vi "Trigger Test Harness.vi"() -> ()   [LabVIEW 2014]
panel:
  in  "Boolean":bool
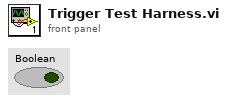
[diagram p1: front panel]
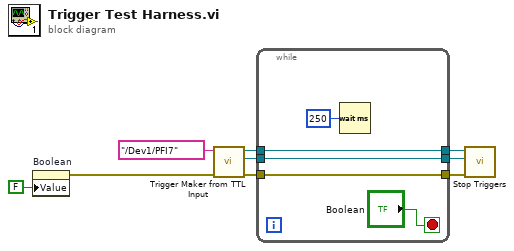
[diagram p0: block diagram]
diagram:
  n1 = property on="Boolean" class="Bool (strict)"("Value"=FALSE ("Boolean")) -> (error out=w1:errorcluster)  [unwired: 2 in, 1 out]
  n2 = call "Trigger Maker from TTL Input.vi"("Error in"=w1, "Master Trigger In from Laser (TTL)"=tag "/Dev1/PFI7") -> ("error out"=w8:errorcluster, "Alazar Task"=w7:refnum<k21>, "AFG11000 Task"=w9:refnum<k21>)  [unwired: 7 in]
  n3 = while {
    tunnel: w9 -> [w13]
    tunnel: w8 -> [w12]
    tunnel: w7 -> [w11]
    tunnel: [w13] -> w5
    tunnel: [w12] -> w4
    tunnel: [w11] -> w3
    stop <- "Boolean" stop-if-true
    n4 = Wait (ms)(milliseconds to wait=u32 250) -> ()  [unwired: 1 out]
  }
  n5 = call "Stop Triggers.vi"("Error in"=w4, "Alazar Task"=w3, "AFG11000 Task"=w5) -> ()  [unwired: 8 in, 1 out]
